vi "Trust Actual Server Identity.vi"(8 "error in (no error)":errorcluster, 10 "fingerprint":string, 11 "SSH Client in":refnum<class "Generic Client.lvclass">) -> (0 "error out":errorcluster, 2 "permanent?":bool, 3 "SSH Client out":refnum<class "Generic Client.lvclass">)   [LabVIEW 2020, in "NI_SSH.lvlib" / "Generic Client.lvclass"]
uses:
  <vilib>/net/SSH/Client/Generic/Generic Client.lvclass
  <vilib>/Utility/error.llb/Error Cluster From Error Code.vi
  <vilib>/ErrorRing/Error Ring.xnode
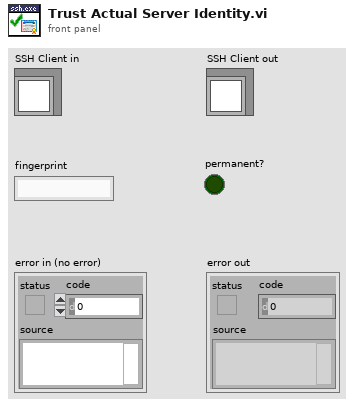
[diagram p1: front panel]
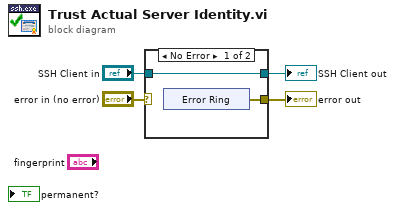
[diagram p0: block diagram]
diagram:
  n1 = case shown="No Error" "error in (no error)" {
    selector: "error in (no error)" -> [_ w12]
    tunnel: [w5 w12] -> w3
    tunnel: [w6 w11] -> w1
    tunnel: "SSH Client in" -> [w6 w11]
    frame No Error {
      n2 = xnode "Error Ring"() -> ("error out"=w5:errorcluster)
    }
    frame Error {
    }
  }
  "error out" <- w3
  "SSH Client out" <- w1
